vi "LWXPS_MultipleAxesPVTLoadToMemory.vi"(6 "LabVIEW error IN":errorcluster, 7 "Trajectory line":string, 8 "Group Name":string, 9 "XPS Reference IN":refnum<k24>) -> (0 "LabVIEW error OUT":errorcluster, 1 "XPS Error String":string, 2 "Returned error code":i32, 3 "XPS Reference OUT":refnum<k24>)   [LabVIEW 2014]
uses:
  D:/XPSQ8_LabView_Library/Development/Source/Dll/Newport.XPS.CommandInterface.dll
  Dll/Newport.XPS.CommandInterface.dll
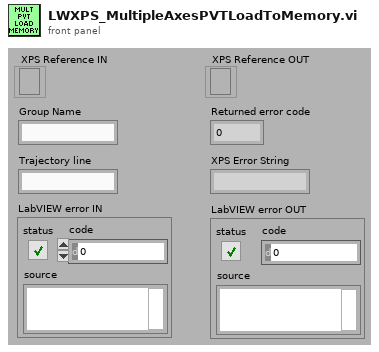
[diagram p1: front panel]
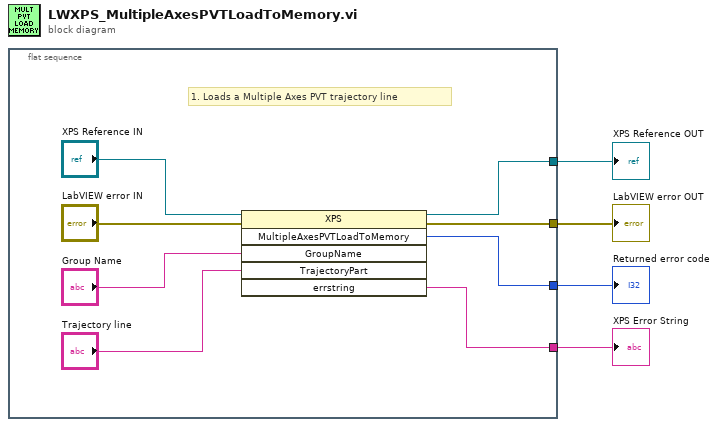
[diagram p0: block diagram]
diagram:
  n1 = flat-sequence {
    tunnel: [w10] -> w4
    tunnel: [w12] -> w3
    tunnel: [w9] -> w2
    tunnel: [w5] -> w1
    frame #0 {
      # "1. Loads a Multiple Axes PVT trajectory line"
      n2 = invoke class="XPS" method="MultipleAxesPVTLoadToMemory"(reference="XPS Reference IN", error in="LabVIEW error IN", "GroupName"="Group Name", "TrajectoryPart"="Trajectory line") -> (reference out=w10:refnum<k24>, error out=w12:errorcluster, "MultipleAxesPVTLoadToMemory"=w9:i32, "errstring"=w5:string)  [unwired: 2 in, 2 out]
    }
  }
  "XPS Reference OUT" <- w4
  "LabVIEW error OUT" <- w3
  "Returned error code" <- w2
  "XPS Error String" <- w1
